vi "KH7008 Set All Channels.vi"(8 "error in (no error)":errorcluster, 10 "Channel Params []":T1[](array[typedef]), 11 "VISA Refnum in":refnum<visa-resource-name>="COM1") -> (0 "error out":errorcluster, 2 "Ch Params [] out":T1[](array[typedef]), 3 "VISA Refnum out":refnum<visa-resource-name>)   [LabVIEW 2019, in "Instrument.KH7008.lvclass"]
uses:
  Instrument.KH7008.lvclass
  typedefs/SetAll-Cluster.ctl
  typedefs/Channel-Enum.ctl
  typedefs/Gain-Enum.ctl
  typedefs/Filter-Enum.ctl
  typedefs/Shunt-Enum.ctl
  typedefs/Coupling-Enum.ctl
  typedefs/Input Configuration-Enum.ctl
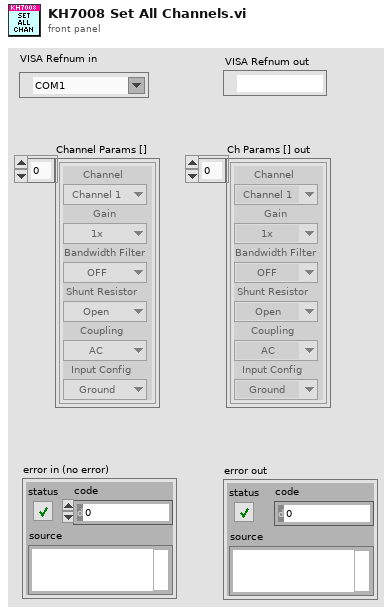
[diagram p1: front panel]
types:
  T1 = typedef "Instrument.KH7008.lvclass/SetAll-Cluster.ctl" = cluster{"Channel":T2, "Gain":T3, "Bandwidth Filter":T4, "Shunt Resistor":T5, "Coupling":T6, "Input Config":T7}
  T2 = typedef "Instrument.KH7008.lvclass/Channel-Enum.ctl" = enum16{"Channel 1", "Channel 2", "Channel 3", "Channel 4", "Channel 5", "Channel 6", "Channel 7", "Channel 8"}
  T3 = typedef "Instrument.KH7008.lvclass/Gain-Enum.ctl" = enum16{"1x", "10x", "100x", "1000x"}
  T4 = typedef "Instrument.KH7008.lvclass/Filter-Enum.ctl" = enum16{"OFF", "ON"}
  T5 = typedef "Instrument.KH7008.lvclass/Shunt-Enum.ctl" = enum16{"Open", "50 Ohms", "500 Ohms", "5k Ohms", "50k Ohms", "10M Ohm"}
  T6 = typedef "Instrument.KH7008.lvclass/Coupling-Enum.ctl" = enum16{"AC", "DC"}
  T7 = typedef "Instrument.KH7008.lvclass/Input Configuration-Enum.ctl" = enum16{"Ground", "SE+ (-gnd)", "SE- (+gnd)", "Differential"}
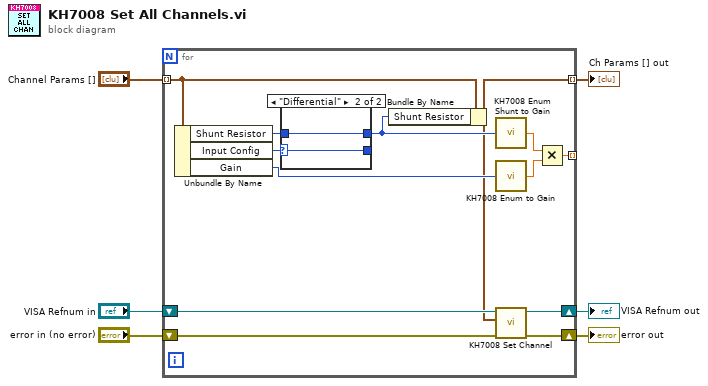
[diagram p0: block diagram]
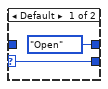
[diagram p2: hidden frame]
diagram:
  n1 = for {
    tunnel: "Channel Params []" -> [w9] mode=indexing
    tunnel: [w19] -> _ mode=indexing
    shift-right: [w18] -> w4
    shift-left: "error in (no error)" -> [w12]
    tunnel: [w8] -> w1 mode=indexing
    shift-right: [w7] -> w2
    shift-left: "VISA Refnum in" -> [w16]
    n2 = Unbundle By Name(w9) -> ("Shunt Resistor"=w15:T5, "Input Config"=w14:T7, "Gain"=w11:T3)
    n3 = case shown="\"Differential\"" w14 {
      selector: w14 -> [w20 w22]
      tunnel: [Shunt-Enum."Open" ("f") w23] -> w10
      tunnel: w15 -> [_ w23]
      tunnel: [w20 w22] -> _
      frame Default {
      }
      frame "Differential" {
      }
    }
    n4 = Bundle By Name(cluster=w9, "Shunt Resistor"=w10) -> (w8:T1)
    n5 = call "KH7008 Enum Shunt to Gain.vi"("Shunt Resistor"=w10) -> ("Gain (V/A)"=w17:dbl)
    n6 = call "KH7008 Enum to Gain.vi"("Gain"=w11) -> ("Gain (x)"=w13:dbl)
    n7 = call "KH7008 Set Channel.vi"("error in (no error)"=w12, "Channel Parameters"=w8, "VISA Refnum in"=w16) -> ("error out"=w18:errorcluster, "VISA Refnum out"=w7:refnum<visa-resource-name>)  [unwired: 7 in]
    n8 = Multiply(x=w17, y=w13) -> (x*y=w19:dbl)
  }
  "error out" <- w4
  "VISA Refnum out" <- w2
  "Ch Params [] out" <- w1
